vi "ConfigTransducer.vi"(2 "configtable":T1 {"CHS"."display" format="%b"}, 3 "Path":path, 4 "root path":path) -> (0 "OK?":bool, 1 "select tr":T4)   [LabVIEW 2011]
uses:
  Instance           1 24Saved   ConfigTransducer .vi
  <vilib>/Analysis/NI_AALPro.lvlib
  singlechtype.ctl
  CHS.ctl
  contable.ctl
panel:
  in  "tablevalue":dbl
  out "TR NO":i32
  in  "type":string(combo) caption="参数类型"
  in  "Auto Calibrate":bool
  in  "CAl":bool
  out "error out 2":errorcluster caption="error out"
  in  "SAVE AS...":bool
  out "error out":errorcluster
  out "Plot Pic":picture caption="通道曲线预览"
  in  "TransducerTable":i32(listbox)
  in  "x End":sgl=10.0 caption="x终止值"
  in  "x Start":sgl=-10.0 caption="x起始值"
  in  "b":sgl caption="b =" format="%05_5f"
  in  "k":sgl=1.0 caption="k =" format="%5_5g"
  in  "TransducerCalc":enum32{"线性", "查表"}(radio) caption="通道换算方法"
  in  "SaveAsDefault":bool
  in  "Load":bool
  in  "OK":bool
  in  "Cancel":bool
  in  "Unit":string(combo) caption="单位"
  in  "Transducer":string caption="传感器名称"
  in  "Insert":bool
  in  "Modify":bool
  in  "Del":bool
  in  "New":bool
  in  "Transducer List":i32(listbox) caption="传感器列表"
  # "传感器参数配置列表"
  # "校准参数方法"
  # "计算公式：y =kx+b"
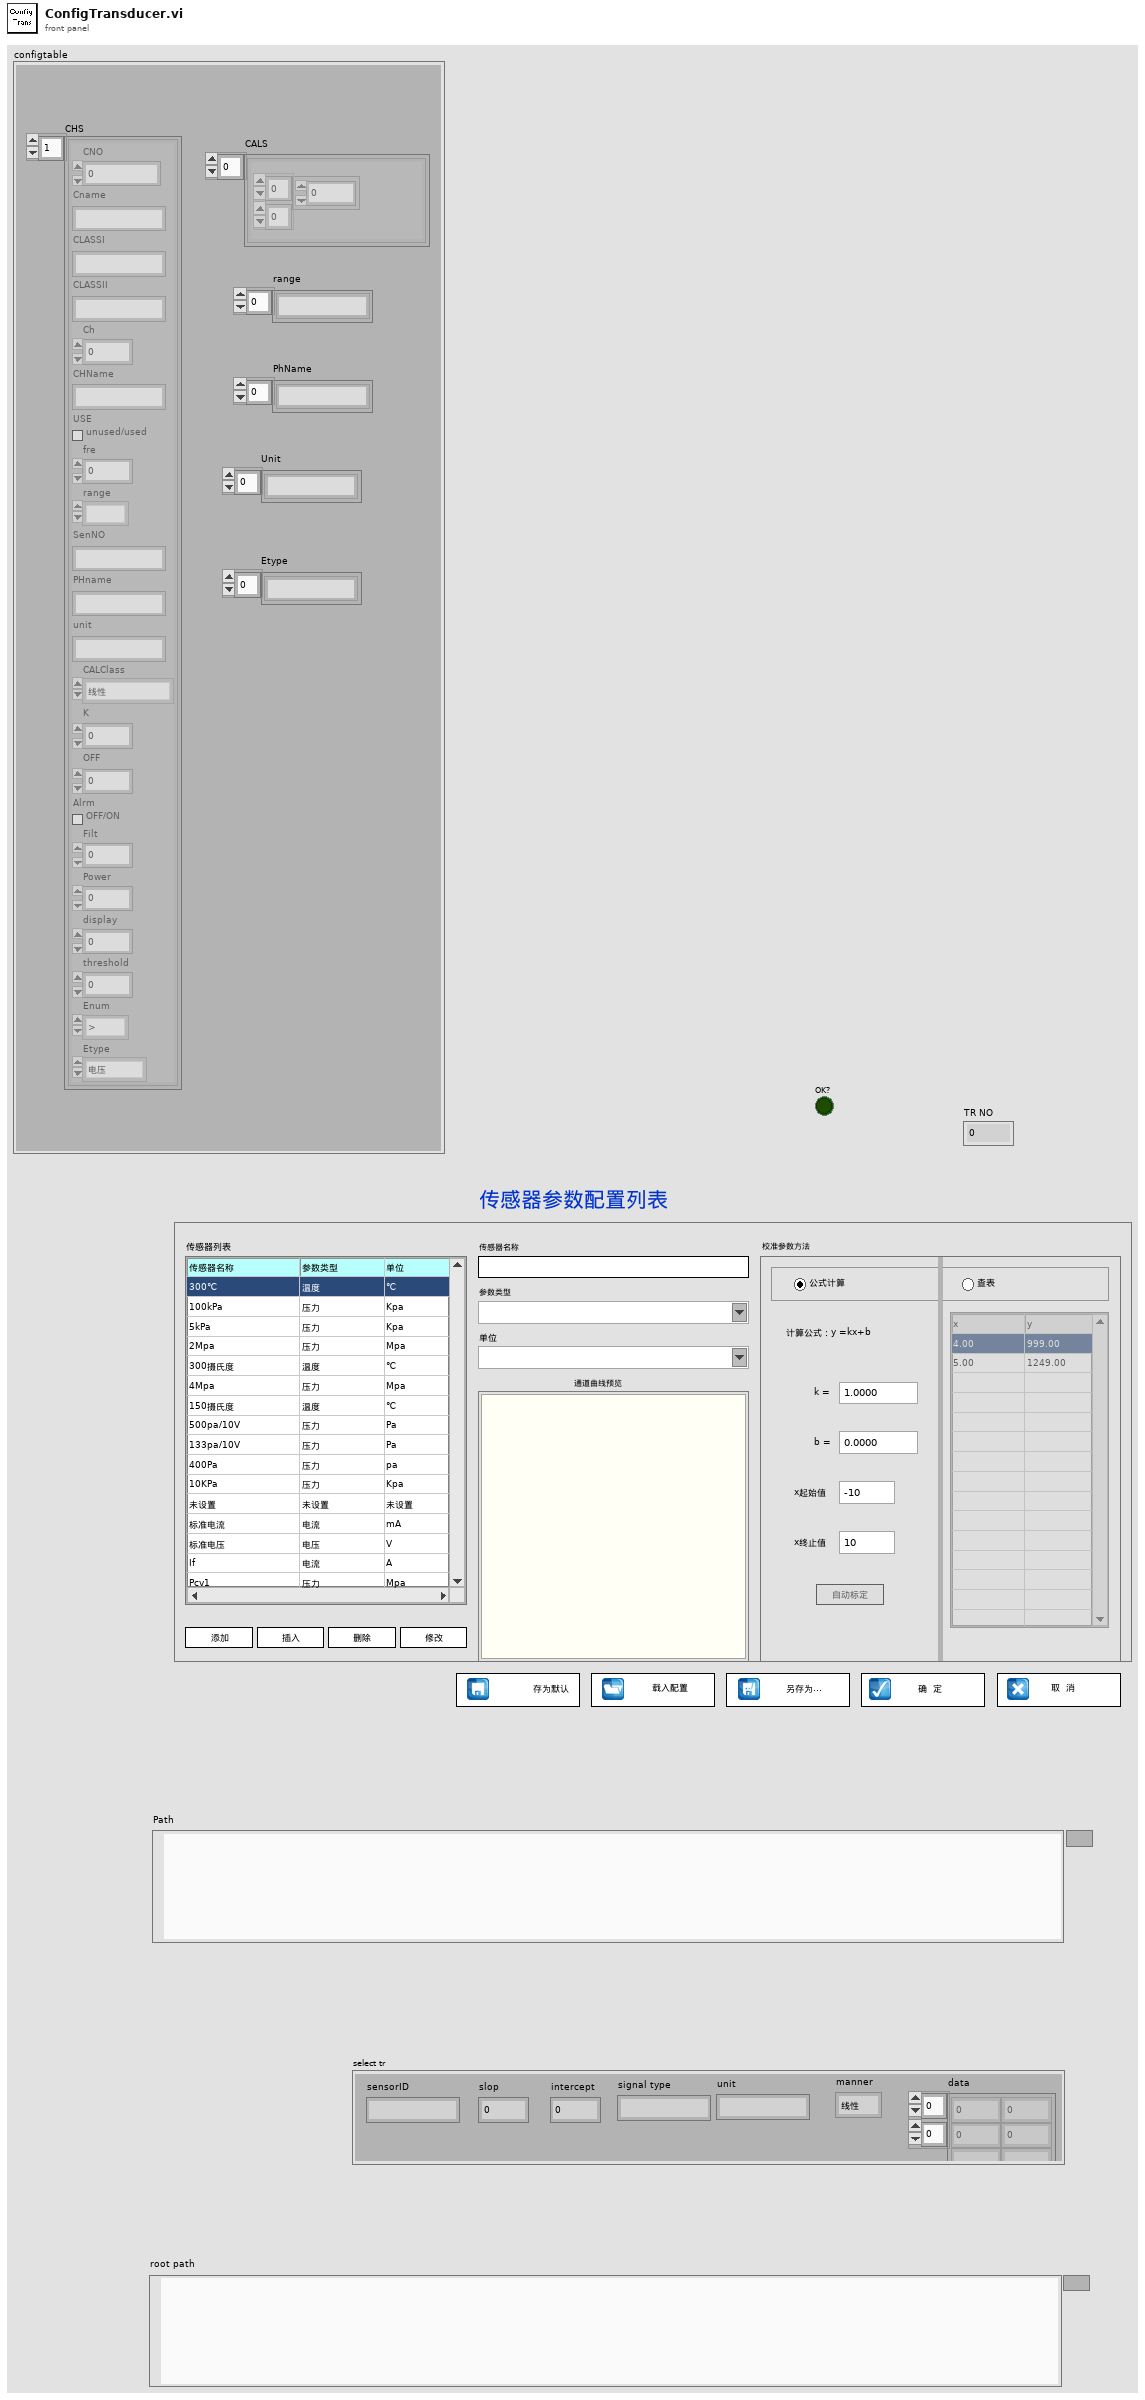
[diagram p1: front panel]
types:
  T1 = typedef "contable.ctl" = cluster{"CHS":T2, "CALS":cluster{"Array":dbl[][]}[], "range":string[], "PhName":string[], "Unit":string[], "Etype":string[]}
  T2 = typedef "CHS.ctl" = T3[]
  T3 = typedef "singlechtype.ctl" = cluster{"CNO":u8, "Cname":string, "CLASSI":string, "CLASSII":string, "Ch":u8, "CHName":string, "USE":bool, "fre":dbl, "range":enum16{""}, "SenNO":string, "PHname":string, "unit":string, "CALClass":enum8{"线性", "查表", "公式"}, "K":dbl, "OFF":dbl, "Alrm":bool, "Filt":dbl, "Power":u8, "display":u8, "threshold ":dbl, "Enum":enum16{">", ">=", "<", "<=", "<>(在范围内）", "><（在范围外）"}, "Etype":enum16{"电压", "电流", "电阻", "热电偶K", "热电偶T"}}
  T4 = cluster{"manner":enum16{"线性", "查表"}, "data":dbl[][], "slop":dbl, "intercept":dbl, "sensorID":string, "signal type":string, "unit":string}
  T5 = cluster{"manner":enum16{"线性", "查表"}, "data":dbl[][], "slop":dbl, "intercept":dbl, "sensorID":string, "signal type":string, "unit":string}[]
  T6 = typedef "LVPoint32TypeDef.ctl" = cluster{"Horizontal":i32, "Vertical":i32}
  T7 = typedef "LVRowAndColumnTypeDef.ctl" = cluster{"Row":i32, "Column":i32}
  T8 = typedef "LVPositionTypeDef.ctl" = cluster{"Left":i32, "Top":i32}
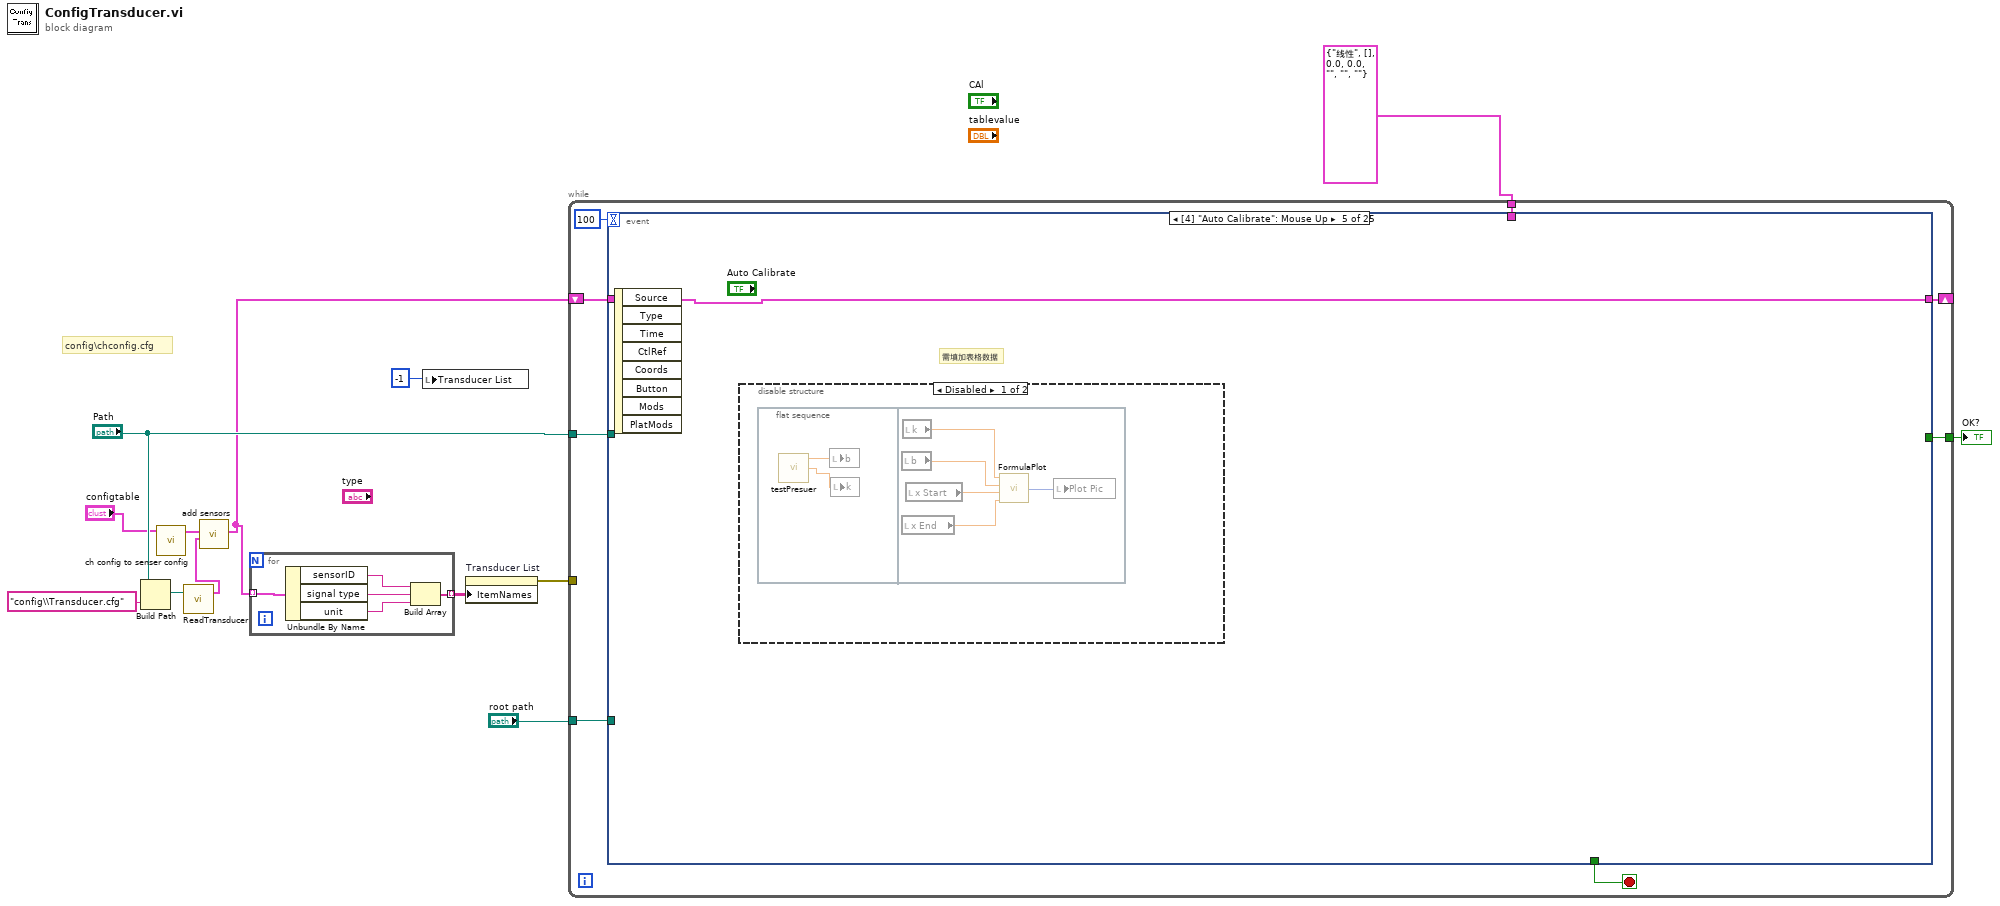
[diagram p0: block diagram]
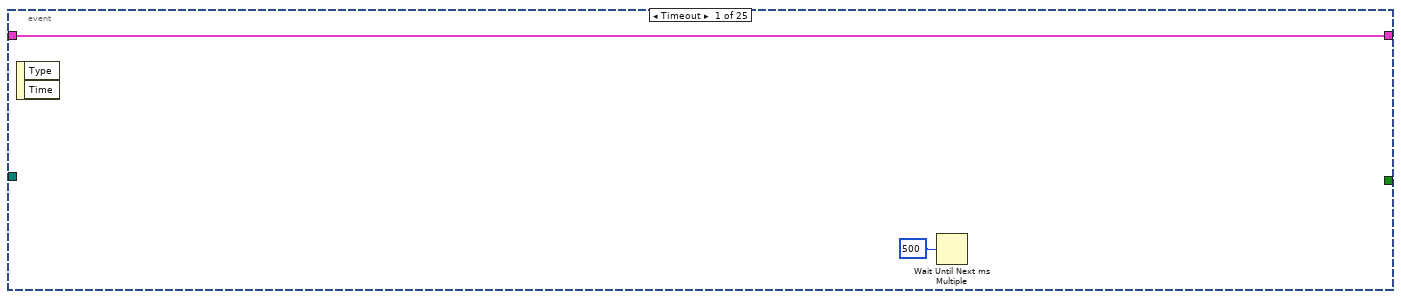
[diagram p2: hidden frame]
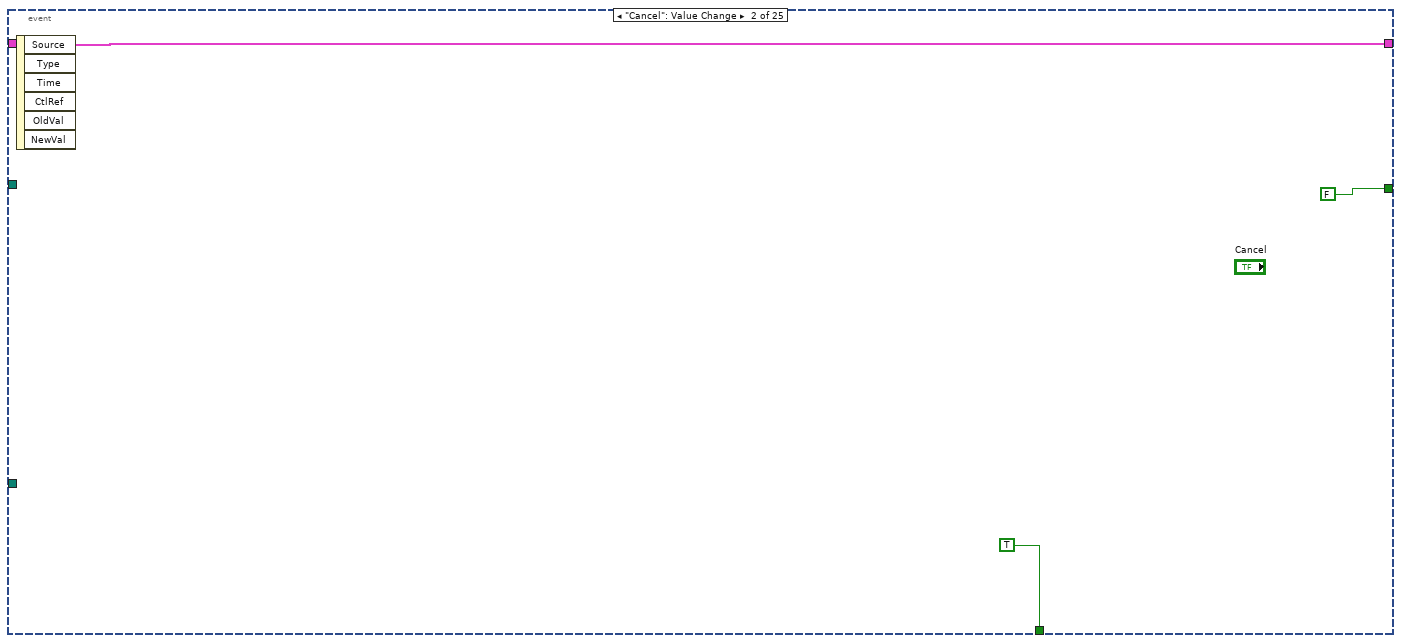
[diagram p3: hidden frame]
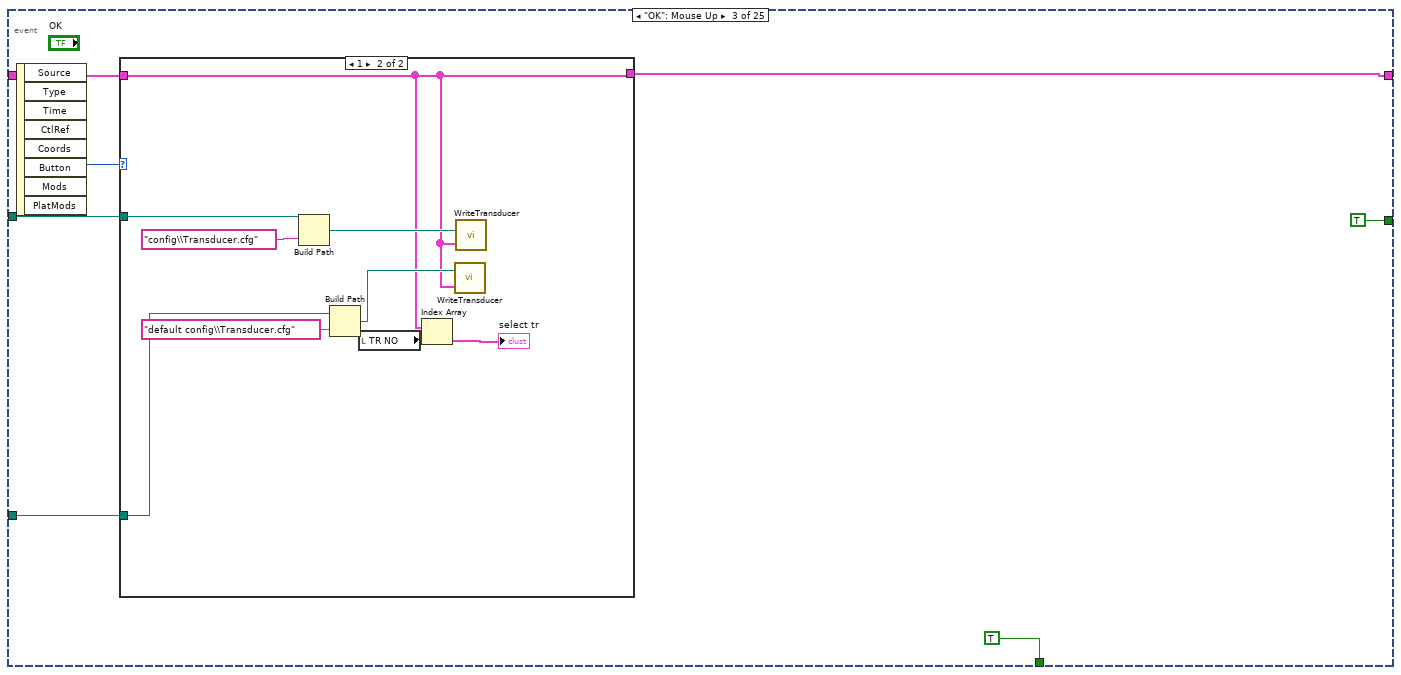
[diagram p4: hidden frame]
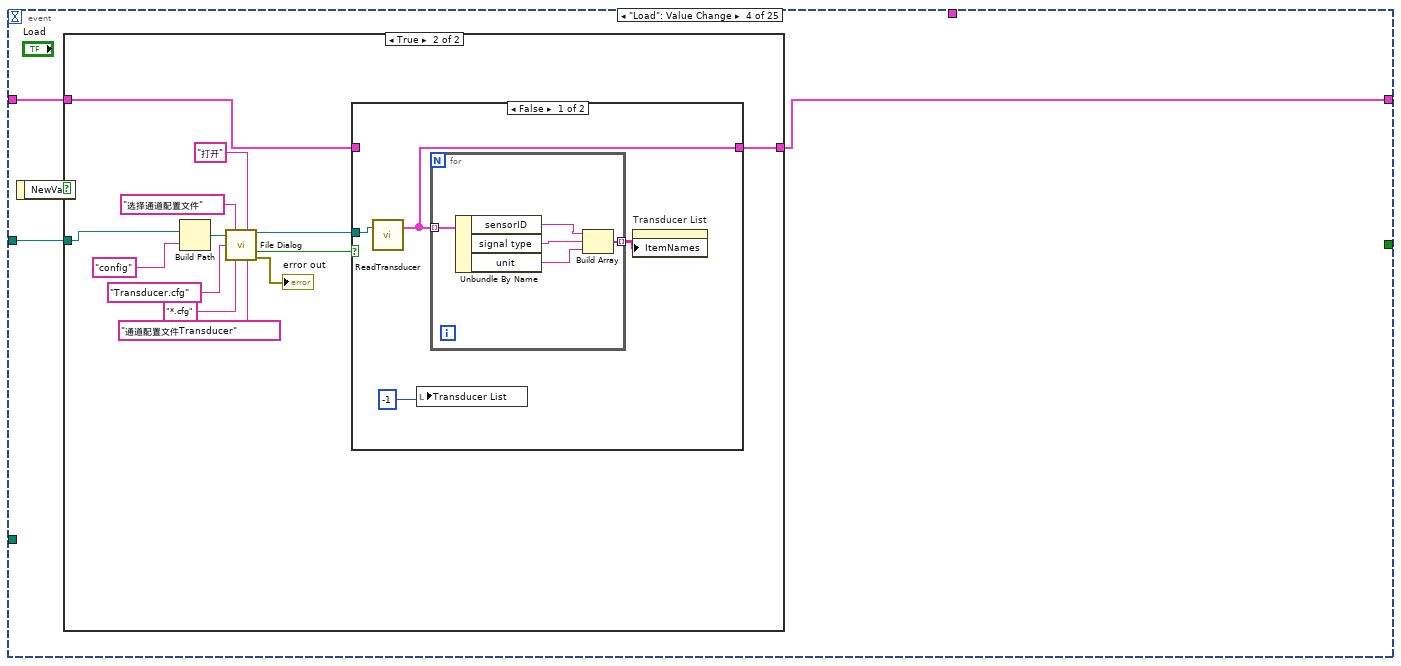
[diagram p6: hidden frame]
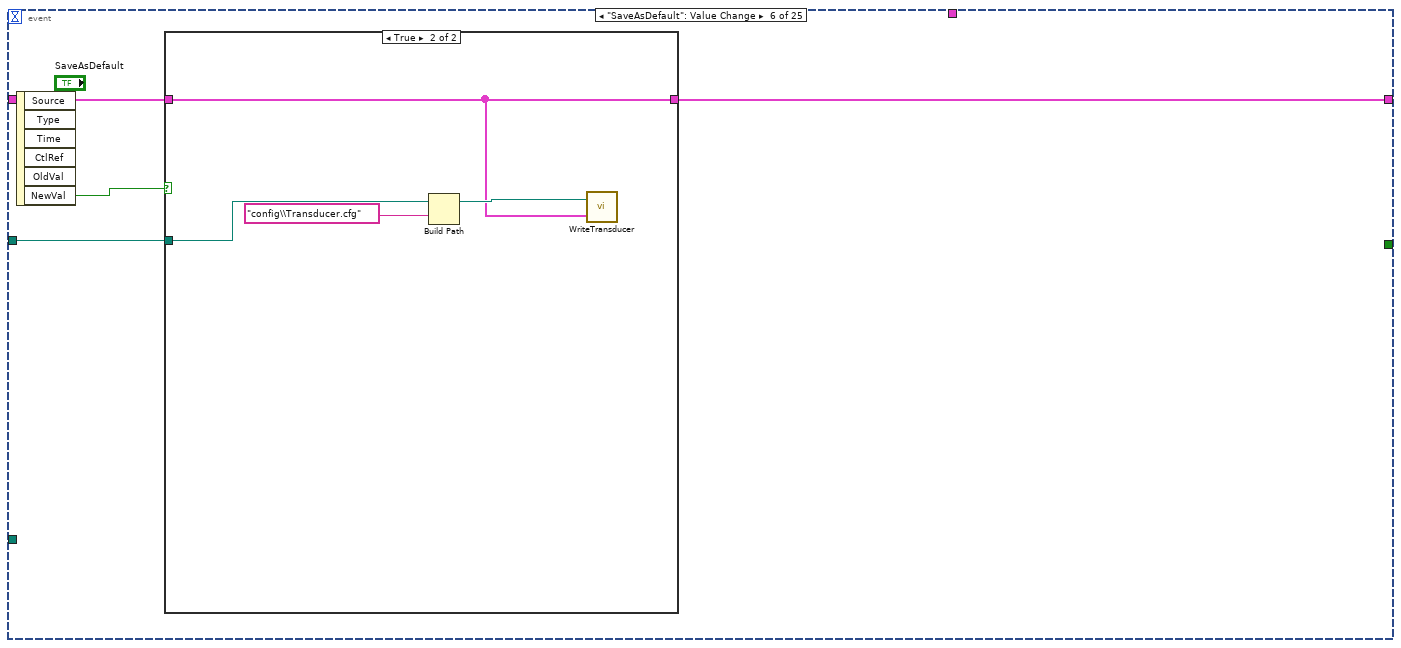
[diagram p10: hidden frame]
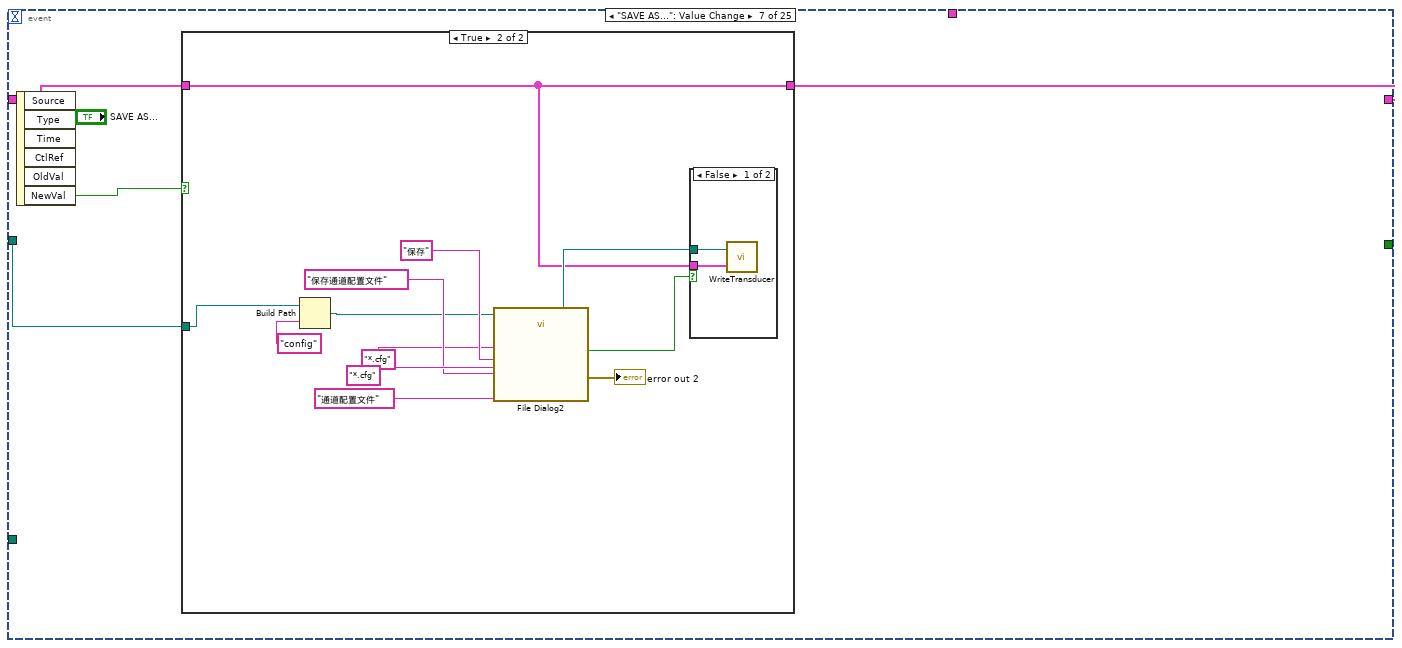
[diagram p12: hidden frame]
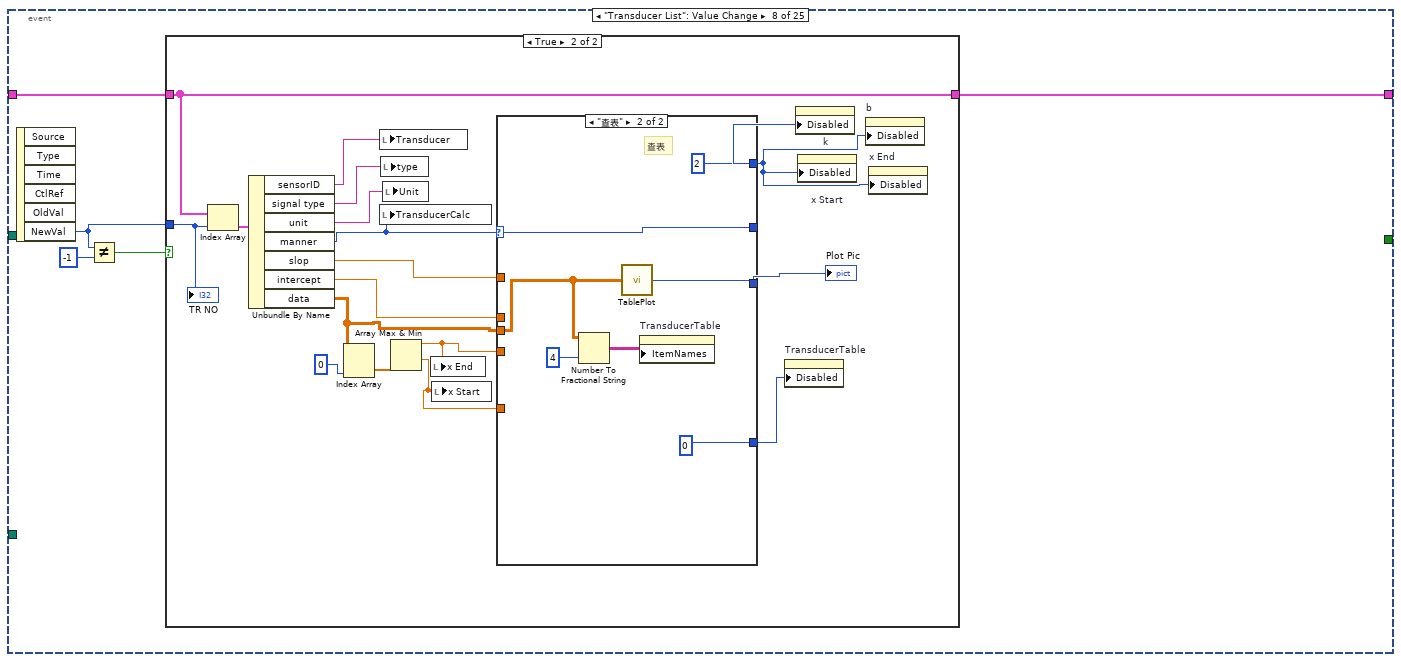
[diagram p15: hidden frame]
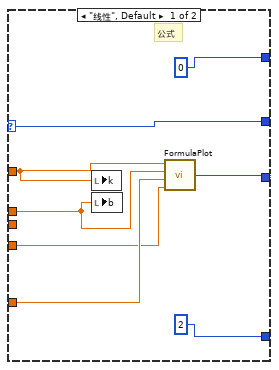
[diagram p17: hidden frame]
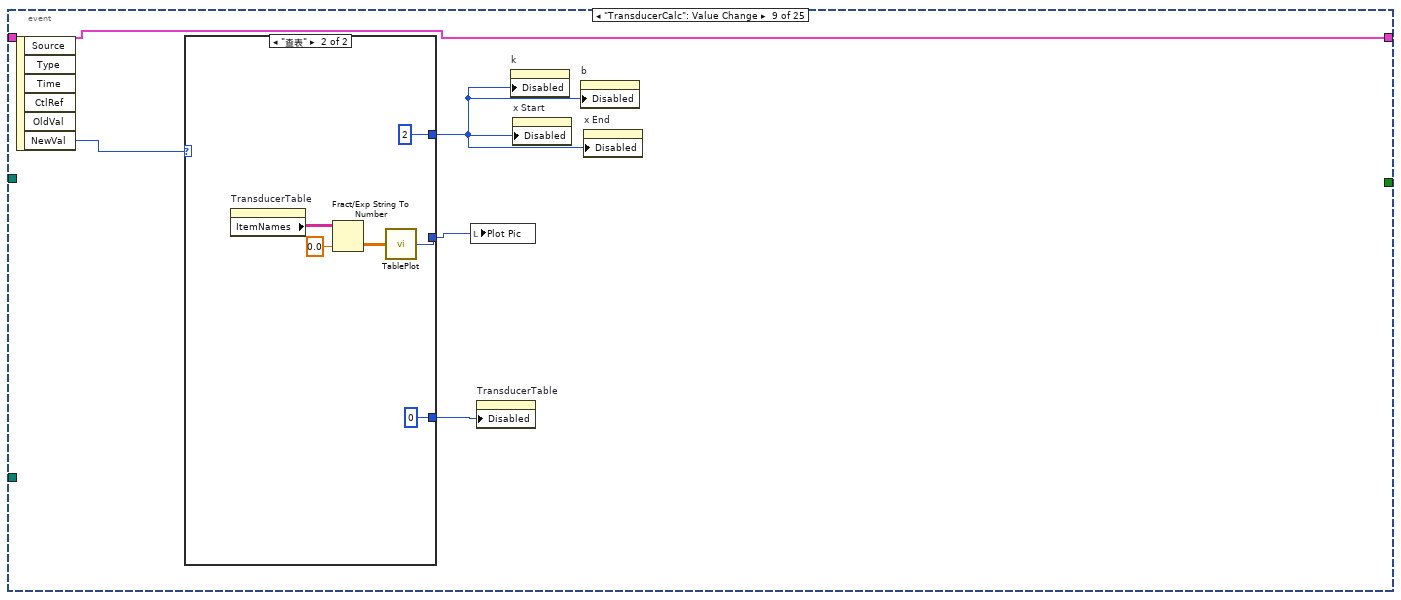
[diagram p18: hidden frame]
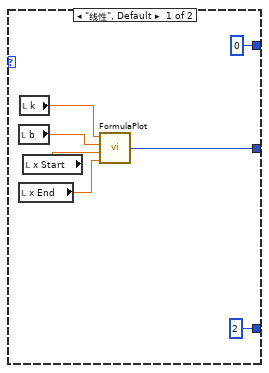
[diagram p19: hidden frame]
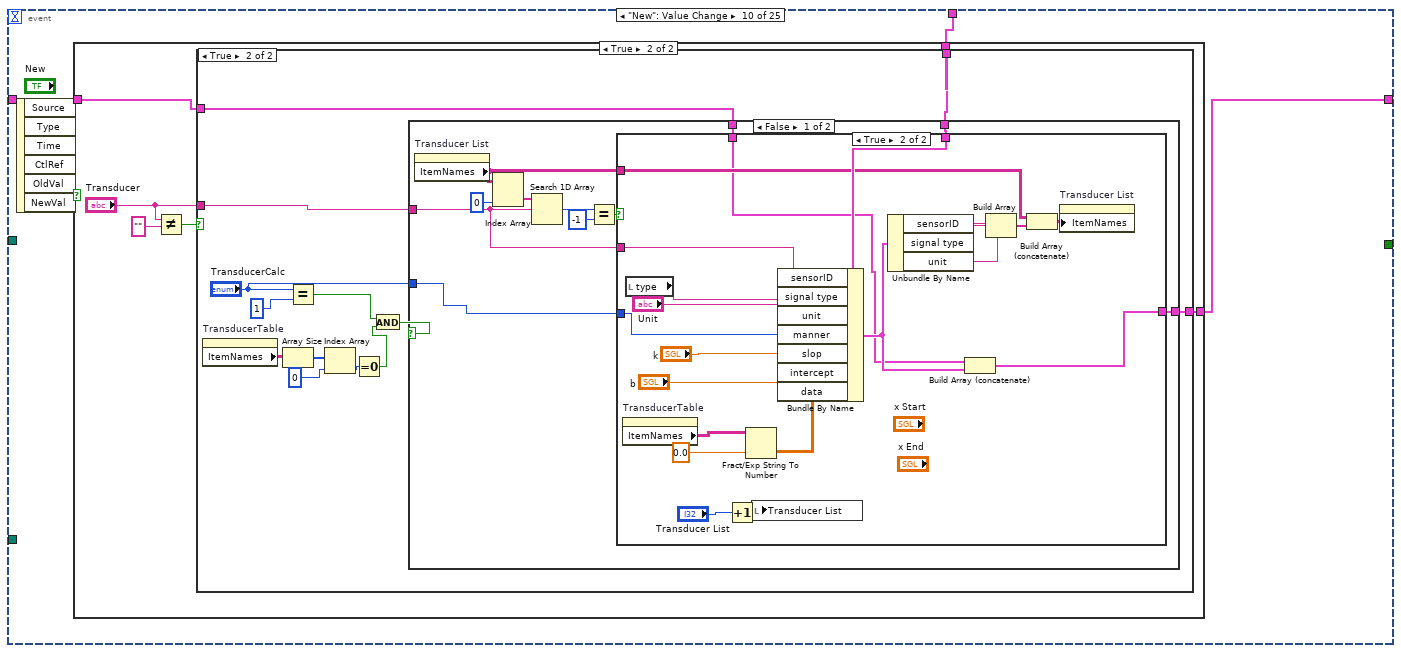
[diagram p20: hidden frame]
diagram:
  # "config\\chconfig.cfg"
  n1 = Build Path(base path="Path", name or relative path="config\\Transducer.cfg") -> (appended path=w9:path)
  n2 = call "ch config to senser config.vi"("configtable"="configtable") -> ("senser out"=w4:T5)  [unwired: 10 out]
  n3 = call "ReadTransducer.vi"("file path"=w9) -> ("sensor"=w2:T5)  [unwired: 1 in, 1 out]
  n4 = call "add sensors.vi"("add sensors"=w2, "sensors"=w4) -> ("sensor out"=w1:T5)  [unwired: 9 out]
  n5 = for {
    tunnel: w1 -> [w18] mode=indexing
    tunnel: [w14] -> w13 mode=indexing
    n6 = Unbundle By Name(w18) -> ("sensorID"=w17:string, "signal type"=w16:string, "unit"=w15:string)
    n7 = Build Array(w17, w16, w15) -> (w14:string[])
  }
  n8 = local write "Transducer List"(-1 ("Transducer List")) -> ()
  n9 = property on="Transducer List" class="MCListbox (strict)"("ItemNames"=w13) -> (error out=w3:errorcluster)  [unwired: 2 in, 1 out]
  n10 = while {
    tunnel: T4 {"manner"=enum."线性", "data"=[], "slop"=0.0, "intercept"=0.0, "sensorID"="", "signal type"="", "unit"=""} ("Sensor") -> [w26]
    tunnel: "Path" -> [w25]
    shift-right: [w22] -> _
    shift-left: w1 -> [w23]
    tunnel: [w20] -> w11
    tunnel: "root path" -> [w19]
    tunnel: w3 -> [_]
    stop <- w24 stop-if-true
    n11 = event shown="[4] \"Auto Calibrate\": Mouse Up" {
      selector: _ -> [_ _ _ _ _ _ _ _ _ _ _ _ _ _ _ _ _ _ _ _ _ _ _ _ _]
      dyn-events: _ -> [_ _ _ _ _ _ _ _ _ _ _ _ _ _ _ _ _ _ _ _ _ _ _ _ _]
      timeout: 100 -> [_ _ _ _ _ _ _ _ _ _ _ _ _ _ _ _ _ _ _ _ _ _ _ _ _]
      tunnel: w26 -> [_ _ _ _ _ _ _ _ _ w171 _ w238 _ w359 _ _ _ _ _ _ _ _ _ _ _]
      tunnel: w25 -> [_ _ w37 w51 _ w87 w96 _ _ _ _ _ _ _ _ _ _ _ _ _ _ _ _ _ _]
      tunnel: [_ TRUE TRUE _ _ _ _ _ _ _ TRUE _ _ _ _ _ _ _ _ _ _ _ _ _ _] -> w24
      tunnel: w23 -> [w28 w30 w35 w49 w77 w86 w95 w114 w151 w169 w234 w236 w312 w357 w433 w435 w459 w464 _ w526 _ w557 w564 w571 w578]
      tunnel: [w28 w30 w34 w50 w77 w85 w94 w113 w151 w170 w234 w237 w311 w358 w433 w434 w459 w464 _ w526 _ w557 w564 w571 w578] -> w22
      tunnel: [_ FALSE TRUE _ _ _ _ _ _ _ _ _ _ _ _ _ _ _ _ _ _ _ _ _ _] -> w20
      tunnel: w19 -> [_ _ w32 _ _ _ _ _ _ _ _ _ _ _ _ _ _ _ _ _ _ _ _ _ _]
      event Timeout {
        n12 = event-data() -> ()  [unwired: 3 out]
        n13 = Wait Until Next ms Multiple(millisecond multiple=u32 500) -> ()  [unwired: 1 out]
      }
      event "Cancel": Value Change {
        n14 = event-data() -> ()  [unwired: 7 out]
      }
      event "OK": Mouse Up {
        n15 = event-data() -> ("Button"=w38:u16)  [unwired: 8 out]
        n16 = case shown="1" w38 {
          tunnel: w37 -> [_ w44]
          tunnel: w35 -> [w39 w40]
          tunnel: [w39 w40] -> w34
          tunnel: w32 -> [_ w42]
          frame 0, Default {
          }
          frame 1 {
            n17 = Build Path(base path=w44, name or relative path="config\\Transducer.cfg" ("pattern (all files)")) -> (appended path=w47:path)
            n18 = Build Path(base path=w42, name or relative path="default config\\Transducer.cfg") -> (appended path=w43:path)
            n19 = local read "TR NO"() -> (w46:i32)
            n20 = Index Array(array=w40, index=w46) -> (element=→"select tr":T4)
            n21 = call "WriteTransducer.vi"("sensor"=w40, "file path"=w43) -> ()
            n22 = call "WriteTransducer.vi"("sensor"=w40, "file path"=w47) -> ()
          }
        }
      }
      event "Load": Value Change {
        n23 = event-data() -> ("NewVal"=w52:bool)  [unwired: 1 out]
        n24 = case shown="True" w52 {
          tunnel: w51 -> [_ w54]
          tunnel: [w53 w56] -> w50
          tunnel: w49 -> [w53 w55]
          frame False {
          }
          frame True {
            n25 = Build Path(base path=w54, name or relative path="config") -> (appended path=w58:path)
            n26 = call "File Dialog"("start path"=w58, "prompt"="选择通道配置文件", "button label"="打开", "default name"="Transducer.cfg" ("pattern (all files)"), "pattern (all files)"="*.cfg", "pattern label"="通道配置文件Transducer" ("default name")) -> ("selected path"=w63:path, "cancelled"=w64:bool, "error out"=→"error out":errorcluster)  [unwired: 1 in, 6 out]
            n27 = case shown="False" w64 {
              tunnel: w63 -> [w70 _]
              tunnel: [w67 w76] -> w56
              tunnel: w55 -> [_ w76]
              frame False {
                n28 = call "ReadTransducer.vi"("file path"=w70) -> ("sensor"=w67:T5)  [unwired: 1 in, 1 out]
                n29 = local write "Transducer List"(-1 ("Transducer List")) -> ()
                n30 = for {
                  tunnel: w67 -> [w75] mode=indexing
                  tunnel: [w71] -> w68 mode=indexing
                  n31 = Unbundle By Name(w75) -> ("sensorID"=w74:string, "signal type"=w73:string, "unit"=w72:string)
                  n32 = Build Array(w74, w73, w72) -> (w71:string[])
                }
                n33 = property on="Transducer List" class="MCListbox (strict)"("ItemNames"=w68) -> ()  [unwired: 2 in, 2 out]
              }
              frame True {
              }
            }
          }
        }
      }
      event "Auto Calibrate": Mouse Up {
        # "需填加表格数据"
        n34 = event-data() -> ()  [unwired: 9 out]
        n35 = disable-structure shown="Disabled" {
          frame Disabled {
            n36 = flat-sequence {
              frame #0 {
                n37 = call "testPresuer.vi"() -> ("b"=w79:dbl, "k"=w78:dbl)  [unwired: 2 out]
                n38 = local write "b"(w79) -> ()
                n39 = local write "k"(w78) -> ()
              }
              frame #1 {
                n40 = local read "b"() -> (w80:sgl)
                n41 = local read "x End"() -> (w84:sgl)
                n42 = local read "k"() -> (w81:sgl)
                n43 = local read "x Start"() -> (w83:sgl)
                n44 = call "FormulaPlot.vi"("X End"=w84, "X Start"=w83, "b"=w80, "k"=w81) -> ("Plot Pic"=w82:picture)
                n45 = local write "Plot Pic"(w82) -> ()
              }
            }
          }
          frame Enabled {
          }
        }
      }
      event "SaveAsDefault": Value Change {
        n46 = event-data() -> ("NewVal"=w88:bool)  [unwired: 6 out]
        n47 = case shown="True" w88 {
          tunnel: w87 -> [_ w90]
          tunnel: w86 -> [w89 w91]
          tunnel: [w89 w91] -> w85
          frame False {
          }
          frame True {
            n48 = Build Path(base path=w90, name or relative path="config\\Transducer.cfg") -> (appended path=w92:path)
            n49 = call "WriteTransducer.vi"("sensor"=w91, "file path"=w92) -> ()
          }
        }
      }
      event "SAVE AS...": Value Change {
        n50 = event-data() -> ("NewVal"=w97:bool)  [unwired: 6 out]
        n51 = case shown="True" w97 {
          tunnel: w96 -> [_ w99]
          tunnel: w95 -> [w98 w100]
          tunnel: [w98 w100] -> w94
          frame False {
          }
          frame True {
            n52 = Build Path(base path=w99, name or relative path="config") -> (appended path=w101:path)
            n53 = call "File Dialog2"("start path"=w101, "prompt"="保存通道配置文件", "button label"="保存", "default name"="*.cfg" ("pattern (all files)"), "pattern (all files)"="*.cfg", "pattern label"="通道配置文件" ("default name")) -> ("selected path"=w105:path, "cancelled"=w104:bool, "error out"=→"error out 2":errorcluster)  [unwired: 1 in, 6 out]
            n54 = case shown="False" w104 {
              tunnel: w105 -> [w111 _]
              tunnel: w100 -> [w112 _]
              frame False {
                n55 = call "WriteTransducer.vi"("sensor"=w112, "file path"=w111) -> ()
              }
              frame True {
              }
            }
          }
        }
      }
      event "Transducer List": Value Change {
        n56 = event-data() -> ("NewVal"=w115:i32)  [unwired: 6 out]
        n57 = Not Equal?(x=w115, y=-1) -> (x != y?=w117:bool)
        n58 = case shown="True" w117 {
          tunnel: w115 -> [_ w135]
          tunnel: w114 -> [w118 w127]
          tunnel: [w118 w127] -> w113
          frame False {
          }
          frame True {
            n59 = Index Array(array=w127, index=w135) -> (element=w134:T4)
            n60 = Unbundle By Name(w134) -> ("sensorID"=w133:string, "signal type"=w128:string, "unit"=w132:string, "manner"=w126:enum16{"线性", "查表"}, "slop"=w125:dbl, "intercept"=w124:dbl, "data"=w120:dbl[][])
            n61 = Index Array(array=w120, index (col)=0 ("disabled index (col)")) -> (element=w123:dbl[])  [unwired: 1 in]
            n62 = local write "Transducer"(w133) -> ()
            n63 = local write "TransducerCalc"(w126) -> ()
            n64 = local write "type"(w128) -> ()
            n65 = local write "Unit"(w132) -> ()
            n66 = Array Max & Min(array=w123) -> (max value=w121:dbl, min value=w122:dbl)  [unwired: 2 out]
            n67 = local write "x End"(w121) -> ()
            n68 = local write "x Start"(w122) -> ()
            n69 = case shown="\"查表\"" w126 {
              selector: w126 -> [w140 w147]
              tunnel: [w143 w148] -> w131
              tunnel: [2 0] -> w129
              tunnel: [0 2] -> w130
              tunnel: [w140 w147] -> _
              tunnel: w125 -> [w139 _]
              tunnel: w124 -> [w138 _]
              tunnel: w122 -> [w137 _]
              tunnel: w121 -> [w136 _]
              tunnel: w120 -> [_ w144]
              frame "线性", Default {
                # "公式"
                n70 = local write "k"(w139) -> ()
                n71 = local write "b"(w138) -> ()
                n72 = call "FormulaPlot.vi"("X End"=w136, "X Start"=w137, "b"=w138, "k"=w139) -> ("Plot Pic"=w143:picture)
              }
              frame "查表" {
                # "查表"
                n73 = Number To Fractional String(number=w144, precision (6)=i16 4) -> (F-format string=w145:string[][])  [unwired: 2 out]
                n74 = call "TablePlot.vi"("表格参数"=w144) -> ("Plot Pic"=w148:picture)
                n75 = property on="TransducerTable" class="MCListbox (strict)"("ItemNames"=w145) -> ()  [unwired: 2 in, 2 out]
              }
            }
            "Plot Pic" <- w131
            n76 = property on="TransducerTable" class="MCListbox (strict)"("Disabled"=w129) -> ()  [unwired: 2 in, 2 out]
            n77 = property on="k" class="DigNum (strict)"("Disabled"=w130) -> ()  [unwired: 2 in, 2 out]
            n78 = property on="x Start" class="DigNum (strict)"("Disabled"=w130) -> ()  [unwired: 2 in, 2 out]
            n79 = property on="b" class="DigNum (strict)"("Disabled"=w130) -> ()  [unwired: 2 in, 2 out]
            n80 = property on="x End" class="DigNum (strict)"("Disabled"=w130) -> ()  [unwired: 2 in, 2 out]
            "TR NO" <- w135
          }
        }
      }
      event "TransducerCalc": Value Change {
        n81 = event-data() -> ("NewVal"=w155:enum32{"线性", "查表"})  [unwired: 6 out]
        n82 = case shown="\"查表\"" w155 {
          tunnel: [w160 w166] -> w153
          tunnel: [0 2] -> w154
          tunnel: [2 0] -> w152
          frame "线性", Default {
            n83 = local read "b"() -> (w156:sgl)
            n84 = local read "x End"() -> (w161:sgl)
            n85 = local read "k"() -> (w157:sgl)
            n86 = local read "x Start"() -> (w162:sgl)
            n87 = call "FormulaPlot.vi"("X End"=w161, "X Start"=w162, "b"=w156, "k"=w157) -> ("Plot Pic"=w160:picture)
          }
          frame "查表" {
            n88 = property on="TransducerTable" class="MCListbox (strict)"() -> ("ItemNames"=w165:string[][])  [unwired: 2 in, 2 out]
            n89 = Fract/Exp String To Number(string=w165, default (0 dbl)=sgl 0.0 ("default (0 I32)")) -> (number=w163:sgl[][])  [unwired: 3 out]
            n90 = call "TablePlot.vi"("表格参数"=w163) -> ("Plot Pic"=w166:picture)
          }
        }
        n91 = local write "Plot Pic"(w153) -> ()
        n92 = property on="TransducerTable" class="MCListbox (strict)"("Disabled"=w152) -> ()  [unwired: 2 in, 2 out]
        n93 = property on="k" class="DigNum (strict)"("Disabled"=w154) -> ()  [unwired: 2 in, 2 out]
        n94 = property on="x Start" class="DigNum (strict)"("Disabled"=w154) -> ()  [unwired: 2 in, 2 out]
        n95 = property on="b" class="DigNum (strict)"("Disabled"=w154) -> ()  [unwired: 2 in, 2 out]
        n96 = property on="x End" class="DigNum (strict)"("Disabled"=w154) -> ()  [unwired: 2 in, 2 out]
      }
      event "New": Value Change {
        n97 = event-data() -> ("NewVal"=w172:bool)  [unwired: 6 out]
        n98 = case shown="True" w172 {
          tunnel: w171 -> [_ w176]
          tunnel: [w173 w175] -> w170
          tunnel: w169 -> [w173 w174]
          frame False {
          }
          frame True {
            n99 = Not Equal?(x="Transducer", y="") -> (x != y?=w178:bool)
            n100 = case shown="True" w178 {
              tunnel: "Transducer" -> [_ w186]
              tunnel: w176 -> [_ w185]
              tunnel: [w180 w183] -> w175
              tunnel: w174 -> [w180 w182]
              frame False {
                n101 = One Button Dialog(message="通道不能为空！") -> ()  [unwired: 2 out]
              }
              frame True {
                n102 = property on="TransducerTable" class="MCListbox (strict)"() -> ("ItemNames"=w194:string[][])  [unwired: 2 in, 2 out]
                n103 = Array Size(array=w194) -> (size(s)=w193:i32[])
                n104 = Equal?(x="TransducerCalc", y=1 ("index")) -> (x = y?=w189:bool)
                n105 = Index Array(array=w193, index=0) -> (element=w191:i32)
                n106 = Equal To 0?(x=w191) -> (x = 0?=w188:bool)
                n107 = And(x=w189, y=w188) -> (x .and. y?=w187:bool)
                n108 = case shown="False" w187 {
                  tunnel: w186 -> [w200 _]
                  tunnel: w185 -> [w199 _]
                  tunnel: "TransducerCalc" -> [w197 _]
                  tunnel: [w196 w232] -> w183
                  tunnel: w182 -> [w195 w232]
                  frame False {
                    n109 = property on="Transducer List" class="MCListbox (strict)"() -> ("ItemNames"=w198:string[][])  [unwired: 2 in, 2 out]
                    n110 = Index Array(array=w198, index (col)=0 ("disabled index (col)")) -> (element=w202:string[])  [unwired: 1 in]
                    n111 = Search 1D Array(1D array=w202, element=w200) -> (index of element=w205:i32)  [unwired: 1 out]
                    n112 = Equal?(x=w205, y=-1) -> (x = y?=w201:bool)
                    n113 = case shown="True" w201 {
                      tunnel: w200 -> [w207 w226]
                      tunnel: w199 -> [_ w231]
                      tunnel: w198 -> [_ w225]
                      tunnel: w197 -> [_ w221]
                      tunnel: [w206 w215] -> w196
                      tunnel: w195 -> [w206 w214]
                      frame False {
                        n114 = Concatenate Strings("“" ("string"), w207, "”已存在，请重新输入。" ("string")) -> (w208:string)
                        n115 = One Button Dialog(message=w208) -> ()  [unwired: 2 out]
                      }
                      frame True {
                        n116 = property on="TransducerTable" class="MCListbox (strict)"() -> ("ItemNames"=w230:string[][])  [unwired: 2 in, 2 out]
                        n117 = local read "type"() -> (w222:string)
                        n118 = Increment(x="Transducer List") -> (x+1=w224:i32)
                        n119 = Fract/Exp String To Number(string=w230, default (0 dbl)=sgl 0.0 ("default (0 I32)")) -> (number=w211:sgl[][])  [unwired: 3 out]
                        n120 = local write "Transducer List"(w224) -> ()
                        n121 = Bundle By Name(cluster=w231, "sensorID"=w226, "signal type"=w222, "unit"="Unit", "manner"=w221, "slop"="k", "intercept"="b", "data"=w211) -> (w220:T4)
                        n122 = Unbundle By Name(w220) -> ("sensorID"=w219:string, "signal type"=w218:string, "unit"=w217:string)
                        n123 = Build Array (concatenate)(w214, w220) -> (w215:T5)
                        n124 = Build Array(w219, w218, w217) -> (w216:string[])
                        n125 = Build Array (concatenate)(w225, w216) -> (w227:string[][])
                        n126 = property on="Transducer List" class="MCListbox (strict)"("ItemNames"=w227) -> ()  [unwired: 2 in, 2 out]
                      }
                    }
                  }
                  frame True {
                    n127 = One Button Dialog(message="表格参数不能为空！") -> ()  [unwired: 2 out]
                  }
                }
              }
            }
          }
        }
      }
      event Panel Close {
        n128 = event-data() -> ()  [unwired: 5 out]
      }
      event "Insert": Value Change {
        n129 = event-data() -> ("NewVal"=w239:bool)  [unwired: 6 out]
        n130 = case shown="True" w239 {
          tunnel: w238 -> [_ w246]
          tunnel: [w240 w242] -> w237
          tunnel: w236 -> [w240 w241]
          frame False {
          }
          frame True {
            n131 = local read "Transducer List"() -> (w243:i32)
            n132 = Not Equal?(x=w243, y=-1) -> (x != y?=w245:bool)
            n133 = case shown="True" w245 {
              tunnel: w246 -> [_ w253]
              tunnel: w243 -> [_ w252]
              tunnel: [w247 w250] -> w242
              tunnel: w241 -> [w247 w249]
              frame False {
                n134 = One Button Dialog(message="请选择想要插入的位置！") -> ()  [unwired: 2 out]
              }
              frame True {
                n135 = local read "Transducer"() -> (w251:string)
                n136 = Not Equal?(x=w251, y="") -> (x != y?=w254:bool)
                n137 = case shown="True" w254 {
                  tunnel: w251 -> [_ w260]
                  tunnel: w253 -> [_ w268]
                  tunnel: w252 -> [_ w267]
                  tunnel: [w256 w259] -> w250
                  tunnel: w249 -> [w256 w258]
                  frame False {
                    n138 = One Button Dialog(message="通道不能为空！") -> ()  [unwired: 2 out]
                  }
                  frame True {
                    n139 = property on="Transducer List" class="MCListbox (strict)"() -> ("ItemNames"=w264:string[][])  [unwired: 2 in, 2 out]
                    n140 = Index Array(array=w264, index (col)=0 ("disabled index (col)")) -> (element=w266:string[])  [unwired: 1 in]
                    n141 = Search 1D Array(1D array=w266, element=w260) -> (index of element=w262:i32)  [unwired: 1 out]
                    n142 = Equal?(x=w262, y=-1) -> (x = y?=w261:bool)
                    n143 = case shown="True" w261 {
                      tunnel: w260 -> [w270 w287]
                      tunnel: w268 -> [_ w286]
                      tunnel: w267 -> [_ w285]
                      tunnel: [w269 w275] -> w259
                      tunnel: w258 -> [w269 w274]
                      frame False {
                        n144 = Concatenate Strings("“" ("string"), w270, "”已存在，请重新输入。" ("string")) -> (w271:string)
                        n145 = One Button Dialog(message=w271) -> ()  [unwired: 2 out]
                      }
                      frame True {
                        n146 = property on="TransducerTable" class="MCListbox (strict)"() -> ("ItemNames"=w279:string[][])  [unwired: 2 in, 2 out]
                        n147 = local read "TransducerCalc"() -> (w277:enum32{"线性", "查表"})
                        n148 = Array Size(array=w279) -> (size(s)=w280:i32[])
                        n149 = Index Array(array=w280, index=0) -> (element=w282:i32)
                        n150 = Equal?(x=w277, y=1 ("index")) -> (x = y?=w278:bool)
                        n151 = Equal To 0?(x=w282) -> (x = 0?=w284:bool)
                        n152 = And(x=w278, y=w284) -> (x .and. y?=w276:bool)
                        n153 = case shown="False" w276 {
                          tunnel: w287 -> [w300 _]
                          tunnel: w277 -> [w306 _]
                          tunnel: w286 -> [w305 _]
                          tunnel: w285 -> [w302 _]
                          tunnel: [w292 w309] -> w275
                          tunnel: w274 -> [w291 w309]
                          frame False {
                            n154 = property on="TransducerTable" class="MCListbox (strict)"() -> ("ItemNames"=w308:string[][])  [unwired: 2 in, 2 out]
                            n155 = local read "type"() -> (w298:string)
                            n156 = local read "Unit"() -> (w299:string)
                            n157 = property on="Transducer List" class="MCListbox (strict)"() -> ("ItemNames"=w304:string[][])  [unwired: 2 in, 2 out]
                            n158 = Increment(x=w302) -> (x+1=w301:i32)
                            n159 = local read "k"() -> (w289:sgl)
                            n160 = local read "b"() -> (w288:sgl)
                            n161 = Fract/Exp String To Number(string=w308, default (0 dbl)=sgl 0.0 ("default (0 I32)")) -> (number=w290:sgl[][])  [unwired: 3 out]
                            n162 = Bundle By Name(cluster=w305, "sensorID"=w300, "signal type"=w298, "unit"=w299, "manner"=w306, "slop"=w289, "intercept"=w288, "data"=w290) -> (w295:T4)
                            n163 = Unbundle By Name(w295) -> ("sensorID"=w294:string, "signal type"=w297:string, "unit"=w296:string)
                            n164 = local write "Transducer List"(w301) -> ()
                            n165 = Insert Into Array "Insert Into Array"(array=w291, index=w301, new element=w295) -> (w292:T5)
                            n166 = Build Array(w294, w297, w296) -> (w293:string[])
                            n167 = Insert Into Array(array=w304, index (row)=w301, new element=w293) -> (w303:string[][])  [unwired: 1 in]
                            n168 = property on="Transducer List" class="MCListbox (strict)"("ItemNames"=w303) -> ()  [unwired: 2 in, 2 out]
                          }
                          frame True {
                            n169 = One Button Dialog(message="表格参数不能为空！") -> ()  [unwired: 2 out]
                          }
                        }
                      }
                    }
                  }
                }
              }
            }
          }
        }
      }
      event "Del": Value Change {
        n170 = event-data() -> ("NewVal"=w313:bool)  [unwired: 6 out]
        n171 = case shown="True" w313 {
          tunnel: w312 -> [w314 w316]
          tunnel: [w314 w315] -> w311
          frame False {
          }
          frame True {
            n172 = local read "Transducer List"() -> (w317:i32)
            n173 = Not Equal?(x=w317, y=-1) -> (x != y?=w318:bool)
            n174 = case shown="True" w318 {
              tunnel: w317 -> [_ w340]
              tunnel: w316 -> [w320 w323]
              tunnel: [w320 w322] -> w315
              frame False {
                n175 = One Button Dialog(message="请选择想要删除的通道！") -> ()  [unwired: 2 out]
              }
              frame True {
                n176 = property on="Transducer List" class="MCListbox (strict)"() -> ("ItemNames"=w339:string[][])  [unwired: 2 in, 2 out]
                n177 = Delete From Array(array=w323, length=1, index=w340) -> (array with subset deleted=w322:T5)  [unwired: 1 out]
                n178 = Delete From Array "Delete From Array"(array=w339, length=1, index (row)=w340) -> (array with subset deleted=w337:string[][])  [unwired: 1 in, 1 out]
                n179 = local read "Transducer List"() -> (w335:i32)
                n180 = property on="Transducer List" class="MCListbox (strict)"("ItemNames"=w337) -> ()  [unwired: 2 in, 2 out]
                n181 = Index Array(array=w322, index=w335) -> (element=w333:T4)
                n182 = Unbundle By Name(w333) -> ("sensorID"=w334:string, "signal type"=w325:string, "unit"=w332:string, "manner"=w327:enum16{"线性", "查表"}, "slop"=w331:dbl, "intercept"=w330:dbl, "data"=w324:dbl[][])
                n183 = local write "Transducer"(w334) -> ()
                n184 = local write "type"(w325) -> ()
                n185 = local write "Unit"(w332) -> ()
                n186 = local write "TransducerCalc"(w327) -> ()
                n187 = case shown="\"查表\"" w327 {
                  tunnel: [w350 w354] -> w329
                  tunnel: [0 0] -> w328
                  tunnel: [2 2] -> w326
                  tunnel: w331 -> [w347 _]
                  tunnel: w330 -> [w346 _]
                  tunnel: w324 -> [w345 w351]
                  frame "线性", Default {
                    n188 = local write "k"(w347) -> ()
                    n189 = Index Array(array=w345, index (col)=0 ("disabled index (col)")) -> (element=w343:dbl[])  [unwired: 1 in]
                    n190 = local write "b"(w346) -> ()
                    n191 = Array Max & Min(array=w343) -> (max value=w341:dbl, min value=w342:dbl)  [unwired: 2 out]
                    n192 = local write "x End"(w341) -> ()
                    n193 = local write "x Start"(w342) -> ()
                    n194 = call "FormulaPlot.vi"("X End"=w341, "X Start"=w342, "b"=w346, "k"=w347) -> ("Plot Pic"=w350:picture)
                  }
                  frame "查表" {
                    n195 = Number To Fractional String(number=w351, precision (6)=i16 2) -> (F-format string=w352:string[][])  [unwired: 2 out]
                    n196 = property on="TransducerTable" class="MCListbox (strict)"("ItemNames"=w352) -> ()  [unwired: 2 in, 2 out]
                    n197 = call "TablePlot.vi"("表格参数"=w351) -> ("Plot Pic"=w354:picture)
                  }
                }
                n198 = property on="TransducerTable" class="MCListbox (strict)"("Disabled"=w326) -> ()  [unwired: 2 in, 2 out]
                n199 = property on="k" class="DigNum (strict)"("Disabled"=w328) -> ()  [unwired: 2 in, 2 out]
                n200 = property on="x Start" class="DigNum (strict)"("Disabled"=w328) -> ()  [unwired: 2 in, 2 out]
                n201 = local write "Plot Pic"(w329) -> ()
                n202 = property on="b" class="DigNum (strict)"("Disabled"=w328) -> ()  [unwired: 2 in, 2 out]
                n203 = property on="x End" class="DigNum (strict)"("Disabled"=w328) -> ()  [unwired: 2 in, 2 out]
              }
            }
          }
        }
      }
      event "Modify": Value Change {
        n204 = event-data() -> ("NewVal"=w360:bool)  [unwired: 6 out]
        n205 = case shown="True" w360 {
          tunnel: w359 -> [_ w364]
          tunnel: [w361 w363] -> w358
          tunnel: w357 -> [w361 w362]
          frame False {
          }
          frame True {
            n206 = local read "Transducer List"() -> (w365:i32)
            n207 = Not Equal?(x=w365, y=-1) -> (x != y?=w366:bool)
            n208 = case shown="True" w366 {
              tunnel: w365 -> [_ w372]
              tunnel: w364 -> [_ w373]
              tunnel: [w368 w371] -> w363
              tunnel: w362 -> [w368 w370]
              frame False {
                n209 = One Button Dialog(message="请选择想要修改的通道配置！") -> ()  [unwired: 2 out]
              }
              frame True {
                n210 = local read "Transducer"() -> (w374:string)
                n211 = Not Equal?(x=w374, y="") -> (x != y?=w375:bool)
                n212 = case shown="True" w375 {
                  tunnel: w374 -> [_ w388]
                  tunnel: w372 -> [_ w387]
                  tunnel: w373 -> [_ w386]
                  tunnel: w372 -> [_ w381]
                  tunnel: [w377 w380] -> w371
                  tunnel: w370 -> [w377 w379]
                  frame False {
                    n213 = One Button Dialog(message="通道不能为空！") -> ()  [unwired: 2 out]
                  }
                  frame True {
                    n214 = property on="Transducer List" class="MCListbox (strict)"() -> ("ItemNames"=w390:string[][])  [unwired: 2 in, 2 out]
                    n215 = Index Array(array=w390, index (col)=0 ("disabled index (col)")) -> (element=w392:string[])  [unwired: 1 in]
                    n216 = Search 1D Array(1D array=w392, element=w388) -> (index of element=w382:i32)  [unwired: 1 out]
                    n217 = Equal?(x=w382, y=w381) -> (x = y?=w383:bool)
                    n218 = Equal?(x=w382, y=-1) -> (x = y?=w385:bool)
                    n219 = Or(x=w385, y=w383) -> (x .or. y?=w384:bool)
                    n220 = case shown="True" w384 {
                      tunnel: w388 -> [w394 w404]
                      tunnel: w387 -> [_ w402]
                      tunnel: w386 -> [_ w401]
                      tunnel: [w393 w400] -> w380
                      tunnel: w379 -> [w393 w399]
                      frame False {
                        n221 = Concatenate Strings("“" ("string"), w394, "”已存在，请重新输入。" ("string")) -> (w395:string)
                        n222 = One Button Dialog(message=w395) -> ()  [unwired: 2 out]
                      }
                      frame True {
                        n223 = property on="TransducerTable" class="MCListbox (strict)"() -> ("ItemNames"=w398:string[][])  [unwired: 2 in, 2 out]
                        n224 = local read "TransducerCalc"() -> (w403:enum32{"线性", "查表"})
                        n225 = Array Size(array=w398) -> (size(s)=w407:i32[])
                        n226 = Index Array(array=w407, index=0) -> (element=w409:i32)
                        n227 = Equal To 0?(x=w409) -> (x = 0?=w411:bool)
                        n228 = Equal?(x=w403, y=1 ("index")) -> (x = y?=w406:bool)
                        n229 = And(x=w406, y=w411) -> (x .and. y?=w405:bool)
                        n230 = case shown="False" w405 {
                          tunnel: w404 -> [w428 _]
                          tunnel: w403 -> [w431 _]
                          tunnel: w402 -> [w427 _]
                          tunnel: w401 -> [w430 _]
                          tunnel: [w417 w432] -> w400
                          tunnel: w399 -> [w416 w432]
                          tunnel: w398 -> [w415 _]
                          frame False {
                            n231 = property on="Transducer List" class="MCListbox (strict)"() -> ("ItemNames"=w426:string[][])  [unwired: 2 in, 2 out]
                            n232 = local read "b"() -> (w413:sgl)
                            n233 = local read "k"() -> (w414:sgl)
                            n234 = local read "type"() -> (w424:string)
                            n235 = Fract/Exp String To Number(string=w415, default (0 dbl)=sgl 0.0 ("default (0 I32)")) -> (number=w412:sgl[][])  [unwired: 3 out]
                            n236 = local read "Unit"() -> (w429:string)
                            n237 = Bundle By Name(cluster=w430, "sensorID"=w428, "signal type"=w424, "unit"=w429, "manner"=w431, "slop"=w414, "intercept"=w413, "data"=w412) -> (w420:T4)
                            n238 = Unbundle By Name(w420) -> ("sensorID"=w419:string, "signal type"=w422:string, "unit"=w421:string)
                            n239 = Replace Array Subset(array=w416, new element=w420, index=w427) -> (w417:T5)
                            n240 = Build Array(w419, w422, w421) -> (w418:string[])
                            n241 = Replace Array Subset(array=w426, new element=w418, index (row)=w427) -> (w425:string[][])  [unwired: 1 in]
                            n242 = property on="Transducer List" class="MCListbox (strict)"("ItemNames"=w425) -> ()  [unwired: 2 in, 2 out]
                          }
                          frame True {
                          }
                        }
                      }
                    }
                  }
                }
              }
            }
          }
        }
      }
      event "CAl": Mouse Up {
        n243 = event-data() -> ()  [unwired: 9 out]
      }
      event Menu Selection (User) {
        n244 = event-data() -> ("ItemTag"=w436:string)  [unwired: 7 out]
        n245 = case shown="\"True\"" w436 {
          tunnel: w435 -> [w437 w439]
          tunnel: [w437 w438] -> w434
          frame "False", Default {
          }
          frame "True" {
            n246 = Not Equal?(x="TransducerTable", y=-1) -> (x != y?=w441:bool)
            n247 = case shown="True" w441 {
              tunnel: "TransducerTable" -> [_ w457]
              tunnel: w439 -> [w443 w446]
              tunnel: [w443 w446] -> w438
              frame False {
                n248 = One Button Dialog(message="请选择想要删除的通道！") -> ()  [unwired: 2 out]
              }
              frame True {
                n249 = property on="TransducerTable" class="MCListbox (strict)"() -> ("ItemNames"=w458:string[][])  [unwired: 2 in, 2 out]
                n250 = Delete From Array(array=w458, length=1, index (row)=w457) -> (array with subset deleted=w453:string[][])  [unwired: 1 in, 1 out]
                n251 = property on="TransducerTable" class="MCListbox (strict)"("ItemNames"=w453) -> ()  [unwired: 2 in, 2 out]
                n252 = Fract/Exp String To Number(string=w453, default (0 dbl)=sgl 0.0 ("default (0 I32)")) -> (number=w445:sgl[][])  [unwired: 3 out]
                n253 = Index Array(array=w445, index (col) #1=0 ("disabled index (col)"), index (col) #2=1 ("index (col)")) -> (element #1=w449:sgl[], element #2=w450:sgl[])  [unwired: 2 in]
                n254 = call "TablePlot.vi"("表格参数"=w445) -> ("Plot Pic"=w454:picture)
                n255 = local write "Plot Pic"(w454) -> ()
                n256 = call <vilib>:"Linear Fit.vi"("Y"=w450, "X"=w449) -> ("slope"=w448:dbl, "intercept"=w447:dbl)  [unwired: 4 in, 8 out]
                n257 = local write "b"(w447) -> ()
                n258 = local write "k"(w448) -> ()
              }
            }
          }
        }
      }
      event "TransducerTable": Shortcut Menu Activation? {
        n259 = event-data() -> ("MenuRef"=w463:refnum<k9>)  [unwired: 7 out]
        n260 = Delete Menu Items(9:w463) -> (3:w462:refnum<k9>)  [unwired: 1 in, 3 out]
        n261 = Insert Menu Items(7:string[] ["SQL_INSERT", "SQL_DEL"] ("item tags"), 8:string[] ["插入", "删除"] ("item names"), 9:w462) -> ()  [unwired: 1 in, 5 out]
        n262 = event-data() -> ()  [unwired: 1 in, 2 out]
      }
      event "TransducerTable": Shortcut Menu Selection (User) {
        n263 = event-data() -> ("CtlRef"=w465:refnum<vi>, "ItemTag"=w466:string)  [unwired: 7 out]
        n264 = case shown="\"SQL_INSERT\"" w466 {
          tunnel: w465 -> [_ w490 w505]
          frame "False", Default {
          }
          frame "SQL_INSERT" {
            n265 = property class="MCListbox (strict)"(reference=w490) -> (reference out=w478:refnum<vi>, "Value"=w481:i32, "ItemNames"=w489:string[][])  [unwired: 1 in, 1 out]
            n266 = Decrement(x=w481) -> (x-1=w488:i32)
            n267 = Index Array(array=w489, index (row) #1=w481, index (row) #2=w488) -> (element #1=w487:string[], element #2=w486:string[])  [unwired: 2 in]
            n268 = Fract/Exp String To Number(string=w487) -> (number=w485:dbl[])  [unwired: 4 out]
            n269 = Fract/Exp String To Number(string=w486) -> (number=w484:dbl[])  [unwired: 4 out]
            n270 = Add(x=w485, y=w484) -> (x+y=w483:dbl[])
            n271 = Divide(x=w483, y=2.0) -> (x/y=w480:dbl[])
            n272 = Number To Fractional String(number=w480, precision (6)=i16 4) -> (F-format string=w479:string[])  [unwired: 2 out]
            n273 = Insert Into Array(array=w489, index (row)=w481, new element=w479) -> (w468:string[][])  [unwired: 1 in]
            n274 = property class="MCListbox (strict)"(reference=w478, "ItemNames"=w468) -> ()  [unwired: 1 in, 2 out]
            n275 = Fract/Exp String To Number(string=w468, default (0 dbl)=sgl 0.0 ("default (0 I32)")) -> (number=w471:sgl[][])  [unwired: 3 out]
            n276 = Index Array(array=w471, index (col) #1=0 ("disabled index (col)"), index (col) #2=1 ("index (col)")) -> (element #1=w472:sgl[], element #2=w473:sgl[])  [unwired: 2 in]
            n277 = call "TablePlot.vi"("表格参数"=w471) -> ("Plot Pic"=w476:picture)
            n278 = local write "Plot Pic"(w476) -> ()
            n279 = call <vilib>:"Linear Fit.vi"("Y"=w473, "X"=w472) -> ("slope"=w470:dbl, "intercept"=w469:dbl)  [unwired: 4 in, 8 out]
            n280 = local write "b"(w469) -> ()
            n281 = local write "k"(w470) -> ()
          }
          frame "SQL_DEL" {
            n282 = property class="MCListbox (strict)"(reference=w505) -> (reference out=w504:refnum<vi>, "Value"=w502:i32, "ItemNames"=w503:string[][])  [unwired: 1 in, 1 out]
            n283 = Delete From Array(array=w503, length=1, index (row)=w502) -> (array with subset deleted=w491:string[][])  [unwired: 1 in, 1 out]
            n284 = Fract/Exp String To Number(string=w491, default (0 dbl)=sgl 0.0 ("default (0 I32)")) -> (number=w494:sgl[][])  [unwired: 3 out]
            n285 = property class="MCListbox (strict)"(reference=w504, "ItemNames"=w491) -> ()  [unwired: 1 in, 2 out]
            n286 = Index Array(array=w494, index (col) #1=0 ("disabled index (col)"), index (col) #2=1 ("index (col)")) -> (element #1=w495:sgl[], element #2=w496:sgl[])  [unwired: 2 in]
            n287 = call "TablePlot.vi"("表格参数"=w494) -> ("Plot Pic"=w499:picture)
            n288 = local write "Plot Pic"(w499) -> ()
            n289 = call <vilib>:"Linear Fit.vi"("Y"=w496, "X"=w495) -> ("slope"=w493:dbl, "intercept"=w492:dbl)  [unwired: 4 in, 8 out]
            n290 = local write "b"(w492) -> ()
            n291 = local write "k"(w493) -> ()
          }
        }
      }
      event "TransducerTable": Double Click {
        n292 = event-data() -> ("CtlRef"=w512:refnum<vi>, "Coords"=w507:T6)  [unwired: 8 out]
        n293 = property class="MCListbox (strict)"(reference=w512) -> (reference out=w508:refnum<vi>, "Disabled"=w511:u8)  [unwired: 1 in, 1 out]
        n294 = control-ref of="tablevalue"() -> (w506:refnum<vi>)
        n295 = Equal?(x=w511, y=u8 0) -> (x = y?=w509:bool)
        n296 = case shown="True" w509 {
          tunnel: w508 -> [_ w513]
          tunnel: w507 -> [_ w523]
          tunnel: w506 -> [_ w514]
          frame False {
          }
          frame True {
            n297 = invoke class="MCListbox (strict)" method="Point To Row Column"(reference=w513, "Point"=w523) -> (reference out=w524:refnum<vi>, "CellPosition"=w516:T7)  [unwired: 5 in, 5 out]
            n298 = property class="MCListbox (strict)"(reference=w524, "ActiveCell"=w516) -> ("ActiveCellPos"=w521:T8, "ItemNames"=w522:string[][])  [unwired: 1 in, 2 out]
            n299 = Unbundle(w516) -> ("Row"=w520:i32, "Column"=w519:i32)
            n300 = Index Array(array=w522, index (row)=w520, index (col)=w519) -> (element=w518:string)
            n301 = Fract/Exp String To Number(string=w518) -> (number=w517:dbl)  [unwired: 4 out]
            n302 = property class="DigNum (strict)"(reference=w514, "Position"=w521, "Value"=w517, "Visible"=TRUE) -> ()  [unwired: 1 in, 2 out]
          }
        }
      }
      event "tablevalue": Value Change {
        n303 = event-data() -> ("CtlRef"=w529:refnum<vi>)  [unwired: 4 out]
        n304 = property class="DigNum (strict)"(reference=w529) -> (reference out=w527:refnum<vi>, "Visible"=w528:bool)  [unwired: 1 in, 1 out]
        n305 = control-ref of="TransducerTable"() -> (w525:refnum<vi>)
        n306 = case shown="True" w528 {
          tunnel: w527 -> [_ w545]
          tunnel: w525 -> [_ w544]
          frame False {
          }
          frame True {
            n307 = property class="MCListbox (strict)"(reference=w544) -> (reference out=w543:refnum<vi>, "ItemNames"=w533:string[][], "ActiveCell"=w532:T7)  [unwired: 1 in, 1 out]
            n308 = property class="DigNum (strict)"(reference=w545, "Visible"=FALSE) -> ("Value"=w531:dbl)  [unwired: 1 in, 2 out]
            n309 = call "change tablevalu.vi"("Active Cell"=w532, "Value"=w531, "Item Names"=w533) -> ("tablevalue out"=w530:string[][])  [unwired: 8 out]
            n310 = Fract/Exp String To Number(string=w530, default (0 dbl)=sgl 0.0 ("default (0 I32)")) -> (number=w538:sgl[][])  [unwired: 3 out]
            n311 = property class="MCListbox (strict)"(reference=w543, "ItemNames"=w530) -> ()  [unwired: 1 in, 2 out]
            n312 = Index Array(array=w538, index (col) #1=1 ("disabled index (col)"), index (col) #2=0 ("index (col)")) -> (element #1=w534:sgl[], element #2=w535:sgl[])  [unwired: 2 in]
            n313 = call "TablePlot.vi"("表格参数"=w538) -> ("Plot Pic"=w541:picture)
            n314 = local write "Plot Pic"(w541) -> ()
            n315 = call <vilib>:"Linear Fit.vi"("Y"=w534, "X"=w535) -> ("slope"=w537:dbl, "intercept"=w536:dbl)  [unwired: 4 in, 8 out]
            n316 = local write "b"(w536) -> ()
            n317 = local write "k"(w537) -> ()
          }
        }
      }
      event "tablevalue": Mouse Leave {
        n318 = event-data() -> ("CtlRef"=w549:refnum<vi>)  [unwired: 4 out]
        n319 = property class="DigNum (strict)"(reference=w549) -> (reference out=w548:refnum<vi>, "Key Focus"=w547:bool)  [unwired: 1 in, 1 out]
        n320 = case shown="False" w547 {
          tunnel: w548 -> [w551 _]
          frame False {
            n321 = property class="DigNum (strict)"(reference=w551, "Visible"=FALSE) -> ()  [unwired: 1 in, 2 out]
          }
          frame True {
          }
        }
      }
      event "k": Value Change {
        n322 = event-data() -> ()  [unwired: 7 out]
        n323 = local read "k"() -> (w555:sgl)
        n324 = local read "x End"() -> (w556:sgl)
        n325 = local read "b"() -> (w554:sgl)
        n326 = local read "x Start"() -> (w553:sgl)
        n327 = call "FormulaPlot.vi"("X End"=w556, "X Start"=w553, "b"=w554, "k"=w555) -> ("Plot Pic"=w558:picture)
        n328 = local write "Plot Pic"(w558) -> ()
        n329 = call "pa to list.vi"("x end"=w553, "x start"=w553, "b"=w554, "K"=w555) -> ("F-format string"=w552:string[][])  [unwired: 7 out]
        n330 = property on="TransducerTable" class="MCListbox (strict)"("ItemNames"=w552) -> ()  [unwired: 2 in, 2 out]
      }
      event "b": Value Change {
        n331 = event-data() -> ()  [unwired: 7 out]
        n332 = local read "b"() -> (w561:sgl)
        n333 = local read "x End"() -> (w559:sgl)
        n334 = local read "k"() -> (w562:sgl)
        n335 = local read "x Start"() -> (w560:sgl)
        n336 = call "FormulaPlot.vi"("X End"=w559, "X Start"=w560, "b"=w561, "k"=w562) -> ("Plot Pic"=w565:picture)
        n337 = local write "Plot Pic"(w565) -> ()
        n338 = call "pa to list.vi"("x end"=w560, "x start"=w559, "b"=w561, "K"=w562) -> ("F-format string"=w563:string[][])  [unwired: 7 out]
        n339 = property on="TransducerTable" class="MCListbox (strict)"("ItemNames"=w563) -> ()  [unwired: 2 in, 2 out]
      }
      event "x Start": Value Change {
        n340 = event-data() -> ()  [unwired: 7 out]
        n341 = local read "b"() -> (w568:sgl)
        n342 = local read "x End"() -> (w566:sgl)
        n343 = local read "k"() -> (w569:sgl)
        n344 = local read "x Start"() -> (w567:sgl)
        n345 = call "FormulaPlot.vi"("X End"=w566, "X Start"=w567, "b"=w568, "k"=w569) -> ("Plot Pic"=w572:picture)
        n346 = call "pa to list.vi"("x end"=w566, "x start"=w567, "b"=w568, "K"=w569) -> ("F-format string"=w570:string[][])  [unwired: 7 out]
        n347 = property on="TransducerTable" class="MCListbox (strict)"("ItemNames"=w570) -> ()  [unwired: 2 in, 2 out]
        n348 = local write "Plot Pic"(w572) -> ()
      }
      event "x End": Value Change {
        n349 = event-data() -> ()  [unwired: 7 out]
        n350 = local read "x Start"() -> (w574:sgl)
        n351 = local read "x End"() -> (w573:sgl)
        n352 = local read "k"() -> (w576:sgl)
        n353 = local read "b"() -> (w575:sgl)
        n354 = call "FormulaPlot.vi"("X End"=w573, "X Start"=w574, "b"=w575, "k"=w576) -> ("Plot Pic"=w579:picture)
        n355 = call "pa to list.vi"("x end"=w573, "x start"=w574, "b"=w575, "K"=w576) -> ("F-format string"=w577:string[][])  [unwired: 7 out]
        n356 = property on="TransducerTable" class="MCListbox (strict)"("ItemNames"=w577) -> ()  [unwired: 2 in, 2 out]
        n357 = local write "Plot Pic"(w579) -> ()
      }
    }
  }
  "OK?" <- w11
